vi "Periodic Tasks.vi"(8 "error in":errorcluster) -> ()   [LabVIEW 2019]
doc: "This VI runs in parallel to other tasks. It can contain as many user-defined periodic loops as you need. These can carry out PID or other sorts of timed response."
uses:
  DRIVE_PID_TUNING.ctl
  <vilib>/Rock Robotics/WPI/ThirdParty/JAS_Junk/TrajLib/DIFF_DRIVE_KitBot_WheelSize_ENUM.ctl
  <vilib>/Rock Robotics/WPI/ThirdParty/JAS_Junk/TrajLib/DIFF_DRIVE_ToughBoxMini_GearChoice_ENUM.ctl
  <vilib>/Rock Robotics/WPI/ThirdParty/JAS_Junk/TrajLib/DIFF_DRIVE_ToughBoxMini_MotorChoice_ENUM.ctl
  <vilib>/Rock Robotics/WPI/ThirdParty/JAS_Junk/TrajLib/LinearFilter_ResetToValue.vi
  <vilib>/Rock Robotics/WPI/ThirdParty/JAS_Junk/TrajLib/LinearFilter_Calculate.vi
  <vilib>/Rock Robotics/WPI/ThirdParty/JAS_Junk/TrajLib/MatBuilder_Create.vi
  <vilib>/Rock Robotics/WPI/ThirdParty/JAS_Junk/TrajLib/Rotation_CreateAngle.vi
  <vilib>/Rock Robotics/WPI/ThirdParty/JAS_Junk/TrajLib/Translation_Create.vi
  Robot Global Data.vi
  <vilib>/Rock Robotics/Network Tables/NT Write Number.vi
  <vilib>/Rock Robotics/Network Tables/NT Write Boolean.vi
  <vilib>/Rock Robotics/Network Tables/NT Write Numeric Array.vi
  <vilib>/Rock Robotics/WPI/ThirdParty/JAS_Junk/TrajLib/LinearFilter_MovingAverage.vi
  <vilib>/Rock Robotics/WPI/ThirdParty/JAS_Junk/TrajLib/LinearFilter_LowPassBW1.vi
  <vilib>/Rock Robotics/WPI/ThirdParty/JAS_Junk/TrajLib/LinearFilter_LowPassBW2.vi
  <vilib>/Rock Robotics/WPI/ThirdParty/JAS_Junk/TrajLib/LinearFilter_HighPassBW1.vi
  <vilib>/Rock Robotics/WPI/ThirdParty/JAS_Junk/TrajLib/LinearFilter_HighPassBW2.vi
  <vilib>/Rock Robotics/WPI/ThirdParty/JAS_Junk/TrajLib/Trajectory_Library.lvlib
panel:
  in  "Speed PID":T1={"proportional gain  Kp"=2.2, "Integral Gain Ki"=1.8, "Derivative Gain Kd"=0.0}
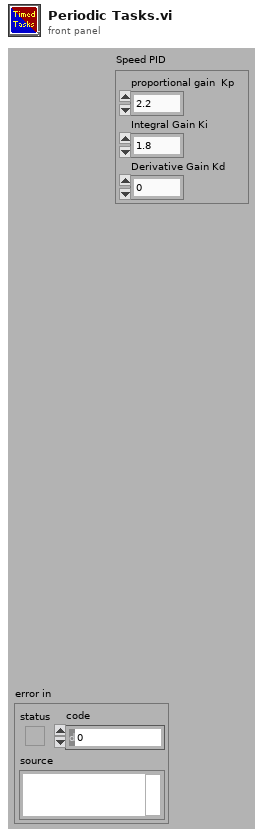
[diagram p1: front panel]
types:
  T1 = typedef "DRIVE_PID_TUNING.ctl" = cluster{"proportional gain  Kp":dbl, "Integral Gain Ki":dbl, "Derivative Gain Kd":dbl}
  T2 = typedef "Trajectory_Library.lvlib/DIFF_DRIVE_ToughBoxMini_MotorChoice_ENUM.ctl" = enum16{"One CIM Per Side", "Two CIM Per Side", "One MiniCIM Per Side", "Two Mini CIM Per Side", "Two Falcon Per Side", "Two NEO Per Side"}
  T3 = typedef "Trajectory_Library.lvlib/DIFF_DRIVE_ToughBoxMini_GearChoice_ENUM.ctl" = enum16{"Ratio_12_75", "Ratio_10_71", "Ratio_8_45", "Ratio_7_31", "Ratio_5_95"}
  T4 = typedef "Trajectory_Library.lvlib/DIFF_DRIVE_KitBot_WheelSize_ENUM.ctl" = enum16{"4 Inch", "6 Inch", "8 Inch", "10 Inch"}
  T5 = typedef "NI_Matrix.lvlib/RealMatrix.ctl" = dbl[][]
  T6 = typedef "Trajectory_Library.lvlib/DIFF_DRIVE_TRAIN_SIM.ctl" = cluster{"m_Plant":T7, "m_X":T5, "m_Y":T5, "m_U":T5, "MeasureStdDev":T5, "m_Motor":T8, "m_OriginalGearing":dbl, "m_CurrentGearing":dbl, "m_WheelRadius_M":dbl, "m_RB":dbl}
  T7 = typedef "Trajectory_Library.lvlib/LINEAR_SYSTEM.ctl" = cluster{"m_A":T5, "m_B":T5, "m_C":T5, "m_D":T5, "States":i32, "Inputs":i32, "Outputs":i32}
  T8 = typedef "Trajectory_Library.lvlib/DCMOTOR.CTL" = cluster{"nominalVoltage_Volts":dbl, "StallTorque_NM":dbl, "StallCurrent_Amps":dbl, "FreeCurrent_Amps":dbl, "FreeSpeed_RadPerSec":dbl, "R_Ohms":dbl, "KvINV_RadPerSecPerVolt":dbl, "Kt_NMPerAmp":dbl, "L_H":dbl, "Jr_KgM2":dbl}
  T9 = typedef "WPI_GyroDevRef.ctl" = cluster{"DevStatus":errorcluster, "Analog Channel":T10, "Gain (VoltsPerDegree/Second)":dbl, "Gyro Type":enum16{"Analog", "XRS450"}, "Handle":i32, "SPI Bus":T11, "Device Found":bool, "Sample Rate":dbl, "Calibrate On Open":bool, "Offset":dbl}
  T10 = typedef "FPGA_AIChannel.ctl" = enum8{"AI 0", "AI 1", "AI 2", "AI 3", "AI MXP 0", "AI MXP 1", "AI MXP 2", "AI MXP 3", "Invalid"}
  T11 = typedef "spi_bus.ctl" = enum16{"SPI On-Board, CS0", "SPI On-Board, CS1", "SPI On-Board, CS2", "SPI On-Board, CS3", "SPI MXP", "Invalid"}
  T12 = typedef "Trajectory_Library.lvlib/POSE2D.ctl" = cluster{"TRANSLATION":T13, "ROTATION":T14}
  T13 = typedef "Trajectory_Library.lvlib/TRANSLATION2D.ctl" = cluster{"X":dbl, "Y":dbl}
  T14 = typedef "Trajectory_Library.lvlib/ROTATION2D.ctl" = cluster{"VALUE":dbl, "COS":dbl, "SIN":dbl}
  T15 = enum16{"Moving Average", "Low Pass 1st Order Butterworth", "Low Pass 2nd Order Butterworth", "High Pass 1st Order Butterworth", "High Pass 2nd Order Butterworth"}
  T16 = typedef "Trajectory_Library.lvlib/SIMPLE_MOTOR_FF.ctl" = cluster{"Ks":dbl, "Kv":dbl, "Ka":dbl}
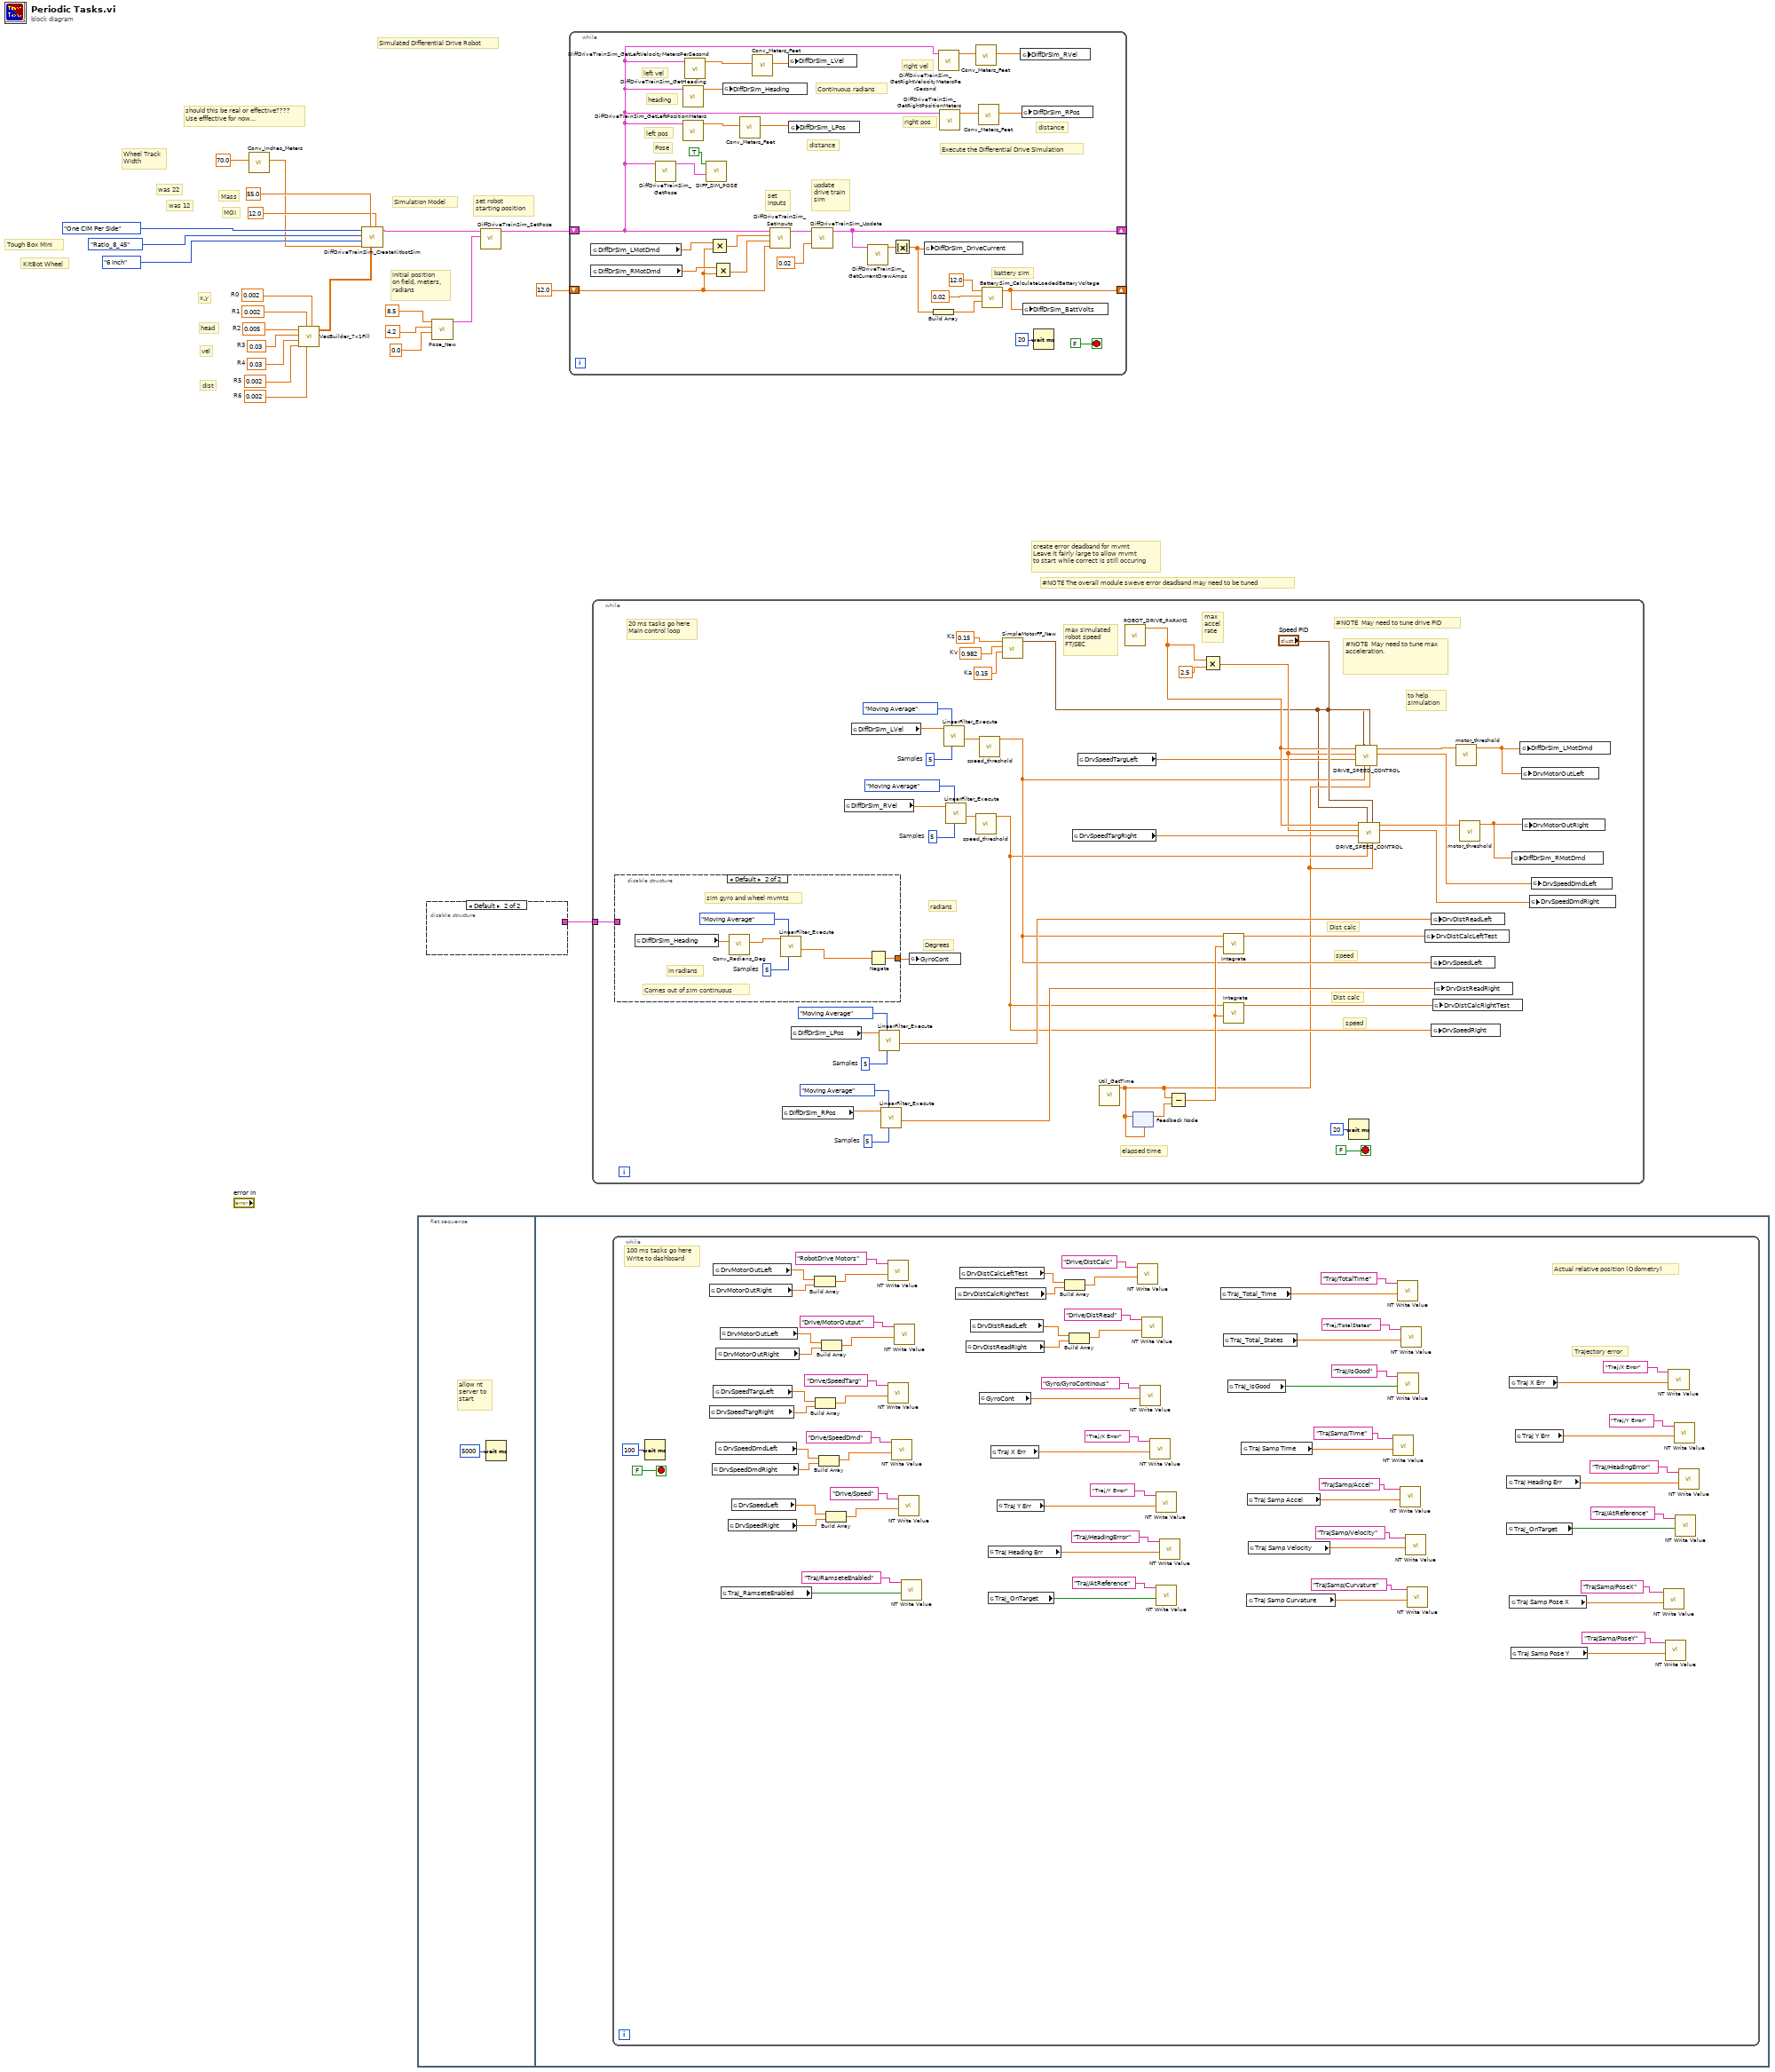
[diagram p0: block diagram]
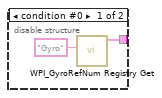
[diagram p2: hidden frame]
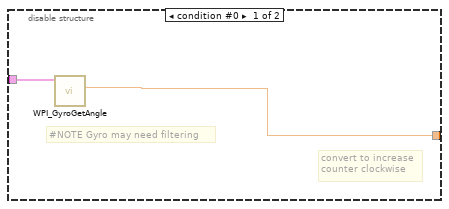
[diagram p3: hidden frame]
diagram:
  w8 = 0.002  # R6
  w7 = 0.002  # R5
  w6 = 0.03  # R4
  w5 = 0.03  # R3
  w4 = 0.005  # R2
  w3 = 0.002  # R1
  w2 = 0.002  # R0
  # "should this be real or effective????\nUse efffective for now..."
  # "dist"
  # "vel"
  # "head"
  # "x,y"
  # "Simulated Differential Drive Robot"
  # "was 12"
  # "set robot\nstarting position"
  # "initial position\non field, meters,\nradians"
  # "was 22"
  # "KitBot Wheel"
  # "Tough Box Mini"
  # "MOI"
  # "Wheel Track\nWidth"
  # "Simulation Model"
  # "Mass"
  # "#NOTE The overall module sweve error deadband may need to be tuned"
  # "create error deadband for mvmt\nLeave it fairly large to allow mvmt\nto start while correct is still occuring"
  n1 = call <vilib>:"Conv_Inches_Meters.vi"("INCH"=70.0 ("ArmLength_M")) -> ("Meters"=w10:dbl)  [unwired: 10 in]
  n2 = call <vilib>:"VecBuilder_7x1Fill.vi"("R0"=w2, "R6"=w8, "R1"=w3, "R5"=w7, "R4"=w6, "R3"=w5, "R2"=w4) -> ("output matrix"=w1:T5)  [unwired: 4 in]
  n3 = call <vilib>:"DiffDriveTrainSim_CreateKitbotSim.vi"("j_KgM2"=12.0 ("Mass_Kg"), "MeasurementStdDev"=w1, "Mass_Kg"=55.0, "TrackWidth_M"=w10, "Wheelsize"=DIFF_DRIVE_KitBot_WheelSize_ENUM."6 Inch" ("Wheel Size"), "ToughBoxMiniGear"=DIFF_DRIVE_ToughBoxMini_GearChoice_ENUM."Ratio_8_45", "ToughBoxMiniMotor"=DIFF_DRIVE_ToughBoxMini_MotorChoice_ENUM."One CIM Per Side") -> ("DiffDriveTrainSim"=w12:T6)  [unwired: 3 in, 1 out]
  n4 = flat-sequence {
    frame #0 {
      # "allow nt\nserver to \nstart"
      n5 = Wait (ms)(milliseconds to wait=u32 5000) -> ()  [unwired: 1 out]
    }
    frame #1 {
      n6 = while {
        stop <- FALSE stop-if-true
        # "Actual relative position (Odometry)"
        # "Trajectory error"
        # "100 ms tasks go here\nWrite to dashboard"
        n7 = Wait (ms)(milliseconds to wait=u32 100) -> ()  [unwired: 1 out]
        n8 = global read "Robot Global Data.vi" "DrvMotorOutRight"() -> (w81:dbl)
        n9 = global read "Robot Global Data.vi" "DrvSpeedTargRight"() -> (w73:dbl)
        n10 = global read "Robot Global Data.vi" "DrvSpeedDmdRight"() -> (w69:dbl)
        n11 = global read "Robot Global Data.vi" "DrvMotorOutLeft"() -> (w82:dbl)
        n12 = global read "Robot Global Data.vi" "DrvSpeedTargLeft"() -> (w74:dbl)
        n13 = global read "Robot Global Data.vi" "DrvMotorOutRight"() -> (w77:dbl)
        n14 = global read "Robot Global Data.vi" "DrvSpeedDmdLeft"() -> (w70:dbl)
        n15 = global read "Robot Global Data.vi" "DrvMotorOutLeft"() -> (w78:dbl)
        n16 = global read "Robot Global Data.vi" "Traj_RamseteEnabled"() -> (w61:bool)
        n17 = global read "Robot Global Data.vi" "DrvSpeedRight"() -> (w65:dbl)
        n18 = global read "Robot Global Data.vi" "DrvSpeedLeft"() -> (w66:dbl)
        n19 = Build Array(w82, w81) -> (w80:dbl[])
        n20 = Build Array(w74, w73) -> (w72:dbl[])
        n21 = Build Array(w70, w69) -> (w68:dbl[])
        n22 = Build Array(w78, w77) -> (w76:dbl[])
        n23 = Build Array(w66, w65) -> (w64:dbl[])
        n24 = call-poly <vilib>:"NT Write Value.vi"("Numeric Array"=w80, "Name"="RobotDrive Motors") -> ()  [unwired: 9 in, 1 out]
        n25 = call-poly <vilib>:"NT Write Value.vi"("Numeric Array"=w72, "Name"="Drive/SpeedTarg") -> ()  [unwired: 9 in, 1 out]
        n26 = call-poly <vilib>:"NT Write Value.vi"("Numeric Array"=w68, "Name"="Drive/SpeedDmd") -> ()  [unwired: 9 in, 1 out]
        n27 = call-poly <vilib>:"NT Write Value.vi"("Numeric Array"=w76, "Name"="Drive/MotorOutput") -> ()  [unwired: 9 in, 1 out]
        n28 = call-poly <vilib>:"NT Write Value.vi"("Numeric Array"=w64, "Name"="Drive/Speed") -> ()  [unwired: 9 in, 1 out]
        n29 = call-poly <vilib>:"NT Write Value.vi"("Boolean"=w61, "Name"="Traj/RamseteEnabled") -> ()  [unwired: 9 in, 1 out]
        n30 = global read "Robot Global Data.vi" "DrvDistCalcRightTest"() -> (w59:dbl)
        n31 = global read "Robot Global Data.vi" "DrvDistCalcLeftTest"() -> (w60:dbl)
        n32 = global read "Robot Global Data.vi" "DrvDistReadRight"() -> (w55:dbl)
        n33 = global read "Robot Global Data.vi" "DrvDistReadLeft"() -> (w56:dbl)
        n34 = global read "Robot Global Data.vi" "GyroCont"() -> (w51:dbl)
        n35 = global read "Robot Global Data.vi" "Traj Heading Err"() -> (w45:dbl)
        n36 = global read "Robot Global Data.vi" "Traj_OnTarget"() -> (w43:bool)
        n37 = global read "Robot Global Data.vi" "Traj X Err"() -> (w49:dbl)
        n38 = global read "Robot Global Data.vi" "Traj Y Err"() -> (w47:dbl)
        n39 = Build Array(w60, w59) -> (w58:dbl[])
        n40 = Build Array(w56, w55) -> (w54:dbl[])
        n41 = call-poly <vilib>:"NT Write Value.vi"("Numeric Array"=w58, "Name"="Drive/DistCalc") -> ()  [unwired: 9 in, 1 out]
        n42 = call-poly <vilib>:"NT Write Value.vi"("Numeric"=w51, "Name"="Gyro/GyroContinous") -> ()  [unwired: 9 in, 1 out]
        n43 = call-poly <vilib>:"NT Write Value.vi"("Numeric Array"=w54, "Name"="Drive/DistRead") -> ()  [unwired: 9 in, 1 out]
        n44 = call-poly <vilib>:"NT Write Value.vi"("Numeric"=w49, "Name"="Traj/X Error") -> ()  [unwired: 9 in, 1 out]
        n45 = call-poly <vilib>:"NT Write Value.vi"("Numeric"=w47, "Name"="Traj/Y Error") -> ()  [unwired: 9 in, 1 out]
        n46 = call-poly <vilib>:"NT Write Value.vi"("Boolean"=w43, "Name"="Traj/AtReference") -> ()  [unwired: 9 in, 1 out]
        n47 = call-poly <vilib>:"NT Write Value.vi"("Numeric"=w45, "Name"="Traj/HeadingError") -> ()  [unwired: 9 in, 1 out]
        n48 = global read "Robot Global Data.vi" "Traj_Total_Time"() -> (w39:dbl)
        n49 = global read "Robot Global Data.vi" "Traj_Total_States"() -> (w38:dbl)
        n50 = global read "Robot Global Data.vi" "Traj_IsGood"() -> (w37:bool)
        n51 = global read "Robot Global Data.vi" "Traj Samp Time"() -> (w33:dbl)
        n52 = global read "Robot Global Data.vi" "Traj Samp Curvature"() -> (w36:dbl)
        n53 = global read "Robot Global Data.vi" "Traj Samp Accel"() -> (w34:dbl)
        n54 = global read "Robot Global Data.vi" "Traj Samp Velocity"() -> (w35:dbl)
        n55 = call-poly <vilib>:"NT Write Value.vi"("Numeric"=w33, "Name"="TrajSamp/Time") -> ()  [unwired: 9 in, 1 out]
        n56 = call-poly <vilib>:"NT Write Value.vi"("Numeric"=w39, "Name"="Traj/TotalTime") -> ()  [unwired: 9 in, 1 out]
        n57 = call-poly <vilib>:"NT Write Value.vi"("Boolean"=w37, "Name"="Traj/IsGood") -> ()  [unwired: 9 in, 1 out]
        n58 = call-poly <vilib>:"NT Write Value.vi"("Numeric"=w34, "Name"="TrajSamp/Accel") -> ()  [unwired: 9 in, 1 out]
        n59 = call-poly <vilib>:"NT Write Value.vi"("Numeric"=w38, "Name"="Traj/TotalStates") -> ()  [unwired: 9 in, 1 out]
        n60 = call-poly <vilib>:"NT Write Value.vi"("Numeric"=w35, "Name"="TrajSamp/Velocity") -> ()  [unwired: 9 in, 1 out]
        n61 = call-poly <vilib>:"NT Write Value.vi"("Numeric"=w36, "Name"="TrajSamp/Curvature") -> ()  [unwired: 9 in, 1 out]
        n62 = global read "Robot Global Data.vi" "Traj Heading Err"() -> (w85:dbl)
        n63 = global read "Robot Global Data.vi" "Traj_OnTarget"() -> (w83:bool)
        n64 = global read "Robot Global Data.vi" "Traj X Err"() -> (w89:dbl)
        n65 = global read "Robot Global Data.vi" "Traj Samp Pose X"() -> (w27:dbl)
        n66 = global read "Robot Global Data.vi" "Traj Samp Pose Y"() -> (w28:dbl)
        n67 = global read "Robot Global Data.vi" "Traj Y Err"() -> (w87:dbl)
        n68 = call-poly <vilib>:"NT Write Value.vi"("Numeric"=w27, "Name"="TrajSamp/PoseX") -> ()  [unwired: 9 in, 1 out]
        n69 = call-poly <vilib>:"NT Write Value.vi"("Numeric"=w28, "Name"="TrajSamp/PoseY") -> ()  [unwired: 9 in, 1 out]
        n70 = call-poly <vilib>:"NT Write Value.vi"("Numeric"=w89, "Name"="Traj/X Error") -> ()  [unwired: 9 in, 1 out]
        n71 = call-poly <vilib>:"NT Write Value.vi"("Numeric"=w87, "Name"="Traj/Y Error") -> ()  [unwired: 9 in, 1 out]
        n72 = call-poly <vilib>:"NT Write Value.vi"("Boolean"=w83, "Name"="Traj/AtReference") -> ()  [unwired: 9 in, 1 out]
        n73 = call-poly <vilib>:"NT Write Value.vi"("Numeric"=w85, "Name"="Traj/HeadingError") -> ()  [unwired: 9 in, 1 out]
      }
    }
  }
  n74 = disable-structure shown="Default" {
    disable-tunnel: [w93 _] -> w23
    frame condition #0 {
      n75 = call <vilib>:"WPI_GyroRefNum Registry Get.vi"("refnum name"="Gyro") -> ("GyroDevRef"=w93:T9)  [unwired: 9 in, 1 out]
    }
    frame condition #1 (active) {
    }
  }
  n76 = call <vilib>:"Pose_New.vi"("Heading"=0.0, "Y"=4.2, "X"=8.5) -> ("out POSe"=w11:T12)  [unwired: 8 in]
  n77 = call <vilib>:"DiffDriveTrainSim_SetPose.vi"("Pose"=w11, "in DiffDriveTrainSim"=w12) -> ("out DiffDriveTrainSim"=w13:T6)  [unwired: 9 in]
  n78 = while {
    shift-right: [w115] -> _
    shift-left: w13 -> [w113]
    shift-right: [w109] -> _
    shift-left: 12.0 ("Voltage") -> [w103]
    stop <- FALSE stop-if-true
    # "Continuous radians"
    # "distance"
    # "distance"
    # "Execute the Differential Drive Simulation"
    # "heading"
    # "left pos"
    # "right pos"
    # "right vel"
    # "left vel"
    # "Pose"
    # "update\ndrive train\nsim"
    # "set\ninputs"
    # "battery sim"
    n79 = global read "Robot Global Data.vi" "DiffDrSim_LMotDmd"() -> (w106:dbl)
    n80 = global read "Robot Global Data.vi" "DiffDrSim_RMotDmd"() -> (w104:dbl)
    n81 = call <vilib>:"DiffDriveTrainSim_GetPose.vi"("DiffDriveTrainSim"=w113) -> ("Pose"=w111:T12)  [unwired: 10 in]
    n82 = call <vilib>:"DiffDriveTrainSim_GetHeading.vi"("DiffDriveTrainSim"=w113) -> ("Heading"=w110:dbl)  [unwired: 10 in]
    n83 = call <vilib>:"DiffDriveTrainSim_GetLeftPositionMeters.vi"("DiffDriveTrainSim"=w113) -> ("LeftPosition_Meters"=w96:dbl)  [unwired: 10 in]
    n84 = call <vilib>:"DiffDriveTrainSim_GetLeftVelocityMetersPerSecond.vi"("DiffDriveTrainSim"=w113) -> ("LeftVelocity_M_Per_Sec"=w98:dbl)  [unwired: 10 in]
    n85 = call "DIFF_SIM_POSE.vi"("in Sim Pose"=w111, "WRITE"=TRUE) -> ()  [unwired: 9 in, 1 out]
    n86 = Multiply(x=w106, y=w103) -> (x*y=w107:dbl)
    n87 = Multiply(x=w104, y=w103) -> (x*y=w105:dbl)
    n88 = global write "Robot Global Data.vi" "DiffDrSim_Heading"(w110) -> ()
    n89 = call <vilib>:"Conv_Meters_Feet.vi"("Meters"=w96) -> ("Feet"=w95:dbl)  [unwired: 10 in]
    n90 = call <vilib>:"Conv_Meters_Feet.vi"("Meters"=w98) -> ("Feet"=w97:dbl)  [unwired: 10 in]
    n91 = call <vilib>:"DiffDriveTrainSim_SetInputs.vi"("BatteryVoltage"=w103, "Right_Volts"=w105, "Left_Volts"=w107, "in DiffDriveTrainSim"=w113) -> ("out DiffDriveTrainSim"=w120:T6)  [unwired: 6 in, 1 out]
    n92 = global write "Robot Global Data.vi" "DiffDrSim_LVel"(w97) -> ()
    n93 = global write "Robot Global Data.vi" "DiffDrSim_LPos"(w95) -> ()
    n94 = call <vilib>:"DiffDriveTrainSim_Update.vi"("dT_Seconds"=0.02, "in DiffDriveTrainSim"=w120) -> ("out DiffDriveTrainSim"=w115:T6)  [unwired: 8 in, 1 out]
    n95 = call <vilib>:"DiffDriveTrainSim_GetCurrentDrawAmps.vi"("DiffDriveTrainSim"=w115) -> ("TotalCurrent_Amps"=w116:dbl)  [unwired: 10 in]
    n96 = Absolute Value(x=w116) -> (abs(x)=w108:dbl)
    n97 = global write "Robot Global Data.vi" "DiffDrSim_DriveCurrent"(w108) -> ()
    n98 = Build Array(w108) -> (w117:dbl[])
    n99 = call <vilib>:"DiffDriveTrainSim_GetRightVelocityMetersPerSecond.vi"("DiffDriveTrainSim"=w113) -> ("RightVel_M_Per_Sec"=w100:dbl)  [unwired: 10 in]
    n100 = call <vilib>:"DiffDriveTrainSim_GetRightPositionMeters.vi"("DiffDriveTrainSim"=w113) -> ("RightPosition_Meters"=w101:dbl)  [unwired: 10 in]
    n101 = call <vilib>:"Conv_Meters_Feet.vi"("Meters"=w100) -> ("Feet"=w99:dbl)  [unwired: 10 in]
    n102 = call <vilib>:"Conv_Meters_Feet.vi"("Meters"=w101) -> ("Feet"=w102:dbl)  [unwired: 10 in]
    n103 = call <vilib>:"BatterySim_CalculateLoadedBatteryVoltage.vi"("Currents"=w117, "Resistance_Ohms"=0.02, "NominalVoltage"=12.0) -> ("Voltage"=w109:dbl)  [unwired: 8 in]
    n104 = global write "Robot Global Data.vi" "DiffDrSim_RVel"(w99) -> ()
    n105 = global write "Robot Global Data.vi" "DiffDrSim_RPos"(w102) -> ()
    n106 = global write "Robot Global Data.vi" "DiffDrSim_BattVolts"(w109) -> ()
    n107 = Wait (ms)(milliseconds to wait=u32 20) -> ()  [unwired: 1 out]
  }
  n108 = while {
    tunnel: w23 -> [w162]
    stop <- FALSE stop-if-true
    w123 = 0.15  # Ks
    w124 = 0.982  # Kv
    w125 = 0.15  # Ka
    w145 = 5  # Samples
    w147 = 5  # Samples
    w151 = 5  # Samples
    w155 = 5  # Samples
    # "Dist calc"
    # "elapsed time"
    # "speed"
    # "speed"
    # "Dist calc"
    # "#NOTE  May need to tune drive PID"
    # "#NOTE  May need to tune max acceleration."
    # "to help\nsimulation"
    # "max simulated\nrobot speed\nFT/SEC"
    # "max\naccel\nrate"
    # "Degrees"
    # "radians"
    # "20 ms tasks go here\nMain control loop"
    n109 = disable-structure shown="Default" {
      disable-tunnel: [w166 w173] -> w163
      disable-tunnel: w162 -> [w167 _]
      frame condition #0 {
        # "#NOTE Gyro may need filtering"
        # "convert to increase\ncounter clockwise"
        n110 = call <vilib>:"WPI_GyroGetAngle.vi"("GyroDevRef"=w167) -> ("Angle"=w166:dbl)  [unwired: 6 in, 4 out]
      }
      frame condition #1 (active) {
        w171 = 5  # Samples
        # "Comes out of sim continuous"
        # "in radians"
        # "sim gyro and wheel mvmts"
        n111 = global read "Robot Global Data.vi" "DiffDrSim_Heading"() -> (w172:dbl)
        n112 = call <vilib>:"Conv_Radians_Deg.vi"("Radians"=w172) -> ("Degrees"=w169:dbl)  [unwired: 10 in]
        n113 = call <vilib>:"LinearFilter_Execute.vi"("Samples"=w171, "Filter Type"=T15."Moving Average", "Input"=w169) -> ("Output"=w168:dbl)  [unwired: 7 in, 1 out]
        n114 = Negate(x=w168) -> (-x=w173:dbl)
      }
    }
    n115 = global read "Robot Global Data.vi" "DiffDrSim_RPos"() -> (w143:dbl)
    n116 = global read "Robot Global Data.vi" "DiffDrSim_LPos"() -> (w141:dbl)
    n117 = global read "Robot Global Data.vi" "DiffDrSim_RVel"() -> (w149:dbl)
    n118 = global read "Robot Global Data.vi" "DiffDrSim_LVel"() -> (w153:dbl)
    n119 = call <vilib>:"LinearFilter_Execute.vi"("Samples"=w147, "Filter Type"=T15."Moving Average", "Input"=w141) -> ("Output"=w140:dbl)  [unwired: 7 in, 1 out]
    n120 = call <vilib>:"LinearFilter_Execute.vi"("Samples"=w145, "Filter Type"=T15."Moving Average", "Input"=w143) -> ("Output"=w142:dbl)  [unwired: 7 in, 1 out]
    n121 = global write "Robot Global Data.vi" "GyroCont"(w163) -> ()
    n122 = call <vilib>:"LinearFilter_Execute.vi"("Samples"=w155, "Filter Type"=T15."Moving Average", "Input"=w153) -> ("Output"=w152:dbl)  [unwired: 7 in, 1 out]
    n123 = call <vilib>:"LinearFilter_Execute.vi"("Samples"=w151, "Filter Type"=T15."Moving Average", "Input"=w149) -> ("Output"=w148:dbl)  [unwired: 7 in, 1 out]
    n124 = call "speed_threshold.vi"("SPEED IN"=w148) -> ("SPEED OUT"=w128:dbl)  [unwired: 10 in]
    n125 = call "speed_threshold.vi"("SPEED IN"=w152) -> ("SPEED OUT"=w129:dbl)  [unwired: 10 in]
    n126 = call <vilib>:"SimpleMotorFF_New.vi"("Ka"=w125, "Kv"=w124, "Ks"=w123) -> ("SIMPLE_MOTOR_FF"=w126:T16)  [unwired: 8 in]
    n127 = global read "Robot Global Data.vi" "DrvSpeedTargRight"() -> (w130:dbl)
    n128 = global read "Robot Global Data.vi" "DrvSpeedTargLeft"() -> (w131:dbl)
    n129 = call <vilib>:"Util_GetTime.vi"() -> ("FPGA_Time_Seconds"=w127:dbl)  [unwired: 10 in, 1 out]
    n130 = call "ROBOT_DRIVE_PARAMS.vi"() -> ("Max Speed Ft/Sec"=w133:dbl)  [unwired: 10 in, 1 out]
    n131 = feedback #1(w127) -> (w157:dbl)
    n132 = feedback-in #1(w127) -> ()
    n133 = Subtract(x=w127, y=w157) -> (x-y=w156:dbl)
    n134 = Multiply(x=w133, y=2.5 ("x")) -> (x*y=w132:dbl)
    n135 = call "Integrate.vi"("Elapsed Sec"=w156, "Rate"=w129) -> ("DIST"=w159:dbl)  [unwired: 9 in]
    n136 = call "Integrate.vi"("Elapsed Sec"=w156, "Rate"=w128) -> ("DIST"=w158:dbl)  [unwired: 9 in]
    n137 = Wait (ms)(milliseconds to wait=u32 20) -> ()  [unwired: 1 out]
    n138 = call "DRIVE_SPEED_CONTROL.vi"("Time_Seconds"=w127, "Speed PID"="Speed PID", "Speed (PV)"=w129, "SIMPLE_MOTOR_FF"=w126, "Speed Target (SP)"=w131, "Max SP Rate"=w132, "Max Speed Ft/Sec"=w133) -> ("SpeedDmd"=w137:dbl, "CO-ControlOutput"=w139:dbl)  [unwired: 1 in, 2 out]
    n139 = call "DRIVE_SPEED_CONTROL.vi"("Time_Seconds"=w127, "Speed PID"="Speed PID", "Speed (PV)"=w128, "SIMPLE_MOTOR_FF"=w126, "Speed Target (SP)"=w130, "Max SP Rate"=w132, "Max Speed Ft/Sec"=w133) -> ("SpeedDmd"=w136:dbl, "CO-ControlOutput"=w138:dbl)  [unwired: 1 in, 2 out]
    n140 = global write "Robot Global Data.vi" "DrvDistCalcLeftTest"(w159) -> ()
    n141 = global write "Robot Global Data.vi" "DrvDistReadLeft"(w140) -> ()
    n142 = global write "Robot Global Data.vi" "DrvSpeedLeft"(w129) -> ()
    n143 = global write "Robot Global Data.vi" "DrvSpeedRight"(w128) -> ()
    n144 = global write "Robot Global Data.vi" "DrvDistCalcRightTest"(w158) -> ()
    n145 = global write "Robot Global Data.vi" "DrvDistReadRight"(w142) -> ()
    n146 = call "motor_threshold.vi"("motor in"=w139) -> ("motor out"=w161:dbl)  [unwired: 10 in]
    n147 = call "motor_threshold.vi"("motor in"=w138) -> ("motor out"=w160:dbl)  [unwired: 10 in]
    n148 = global write "Robot Global Data.vi" "DiffDrSim_RMotDmd"(w160) -> ()
    n149 = global write "Robot Global Data.vi" "DiffDrSim_LMotDmd"(w161) -> ()
    n150 = global write "Robot Global Data.vi" "DrvMotorOutLeft"(w161) -> ()
    n151 = global write "Robot Global Data.vi" "DrvMotorOutRight"(w160) -> ()
    n152 = global write "Robot Global Data.vi" "DrvSpeedDmdRight"(w136) -> ()
    n153 = global write "Robot Global Data.vi" "DrvSpeedDmdLeft"(w137) -> ()
  }
